vi "RocketDrive.vi"(11 "Axes":dbl[](array[numeric])) -> (2 "left setpoint":dbl, 3 "right setpoint":dbl)   [LabVIEW 2019]
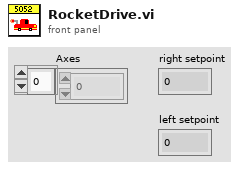
[diagram p1: front panel]
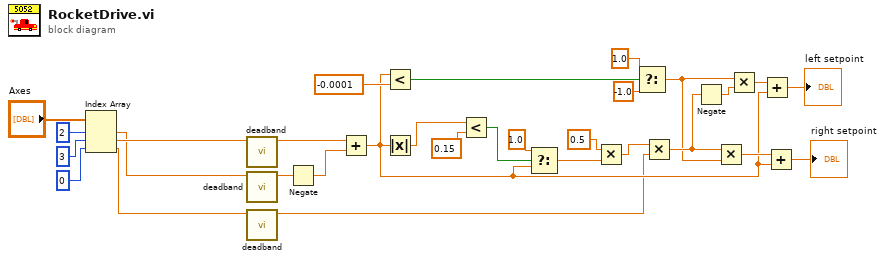
[diagram p0: block diagram]
diagram:
  n1 = Index Array(array="Axes", index #1=2 ("index"), index #2=3 ("index"), index #3=0 ("index")) -> (element #1=w29:dbl, element #2=w30:dbl, element #3=w4:dbl)
  n2 = call "deadband.vi"("Joystick Value"=w30) -> ("Val"=w22:dbl)  [unwired: 10 in]
  n3 = call "deadband.vi"("Joystick Value"=w29) -> ("Val"=w23:dbl)  [unwired: 10 in]
  n4 = call "deadband.vi"("Joystick Value"=w4) -> ("Val"=w1:dbl)  [unwired: 10 in]
  n5 = Negate(x=w23) -> (-x=w21:dbl)
  n6 = Add(x=w22, y=w21) -> (x+y=w9:dbl)
  n7 = Less?(x=w9, y=-0.0001) -> (x < y?=w19:bool)
  n8 = Absolute Value(x=w9) -> (abs(x)=w8:dbl)
  n9 = Less?(x=w8, y=0.15) -> (x < y?=w6:bool)
  n10 = Select(t=1.0, s=w6, f=w9) -> (s? t:f=w5:dbl)
  n11 = Multiply(x=0.5, y=w5) -> (x*y=w2:dbl)
  n12 = Select(t=1.0, s=w19, f=-1.0) -> (s? t:f=w14:dbl)
  n13 = Multiply(x=w2, y=w1) -> (x*y=w16:dbl)
  n14 = Negate(x=w16) -> (-x=w13:dbl)
  n15 = Multiply(x=w16, y=w14) -> (x*y=w15:dbl)
  n16 = Multiply(x=w14, y=w13) -> (x*y=w12:dbl)
  n17 = Add(x=w12, y=w9) -> (x+y=→"left setpoint":dbl)
  n18 = Add(x=w15, y=w9) -> (x+y=→"right setpoint":dbl)
